vi "PathPlanner_GeomUtil_CubicLerp.vi"(6 "T":dbl, 8 "D":T1 {"Y" format="%14.3f"; "X" format="%14.3f"}, 9 "C":T1 {"Y" format="%14.3f"; "X" format="%14.3f"}, 10 "B":T1 {"Y" format="%14.3f"; "X" format="%14.3f"}, 11 "A":T1 {"Y" format="%14.3f"; "X" format="%14.3f"}) -> (3 "Lerp":T1 {"Y" format="%14.3f"; "X" format="%14.3f"})   [LabVIEW 2019, in "PathPlanner24.lvlib"]
doc: "Cubic interpolation between Translation2ds\n \nInputs: \n - a - translation2d - Position 1\n - b - translation2d - Position 2\n - c - translation2d - Position 3\n - t - double - Interpolation factor (0.0-1.0)\n\nOutputs:\n - Lerp - translation2d - Interpolated value"
uses:
  PathPlanner24.lvlib
  <vilib>/Rock Robotics/WPI/ThirdParty/JAS_Junk/TrajLib/TypeDef/TRANSLATION2D.ctl
  <vilib>/Rock Robotics/WPI/ThirdParty/JAS_Junk/TrajLib/Trajectory_Library.lvlib
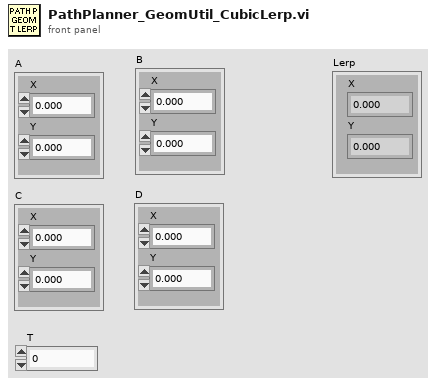
[diagram p1: front panel]
types:
  T1 = typedef "Trajectory_Library.lvlib/TRANSLATION2D.ctl" = cluster{"X":dbl, "Y":dbl}
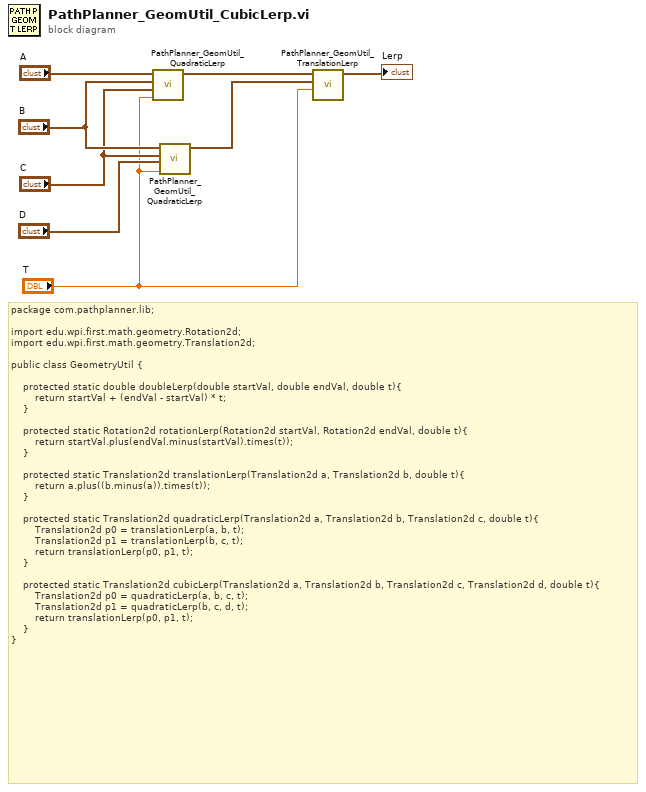
[diagram p0: block diagram]
diagram:
  # "package com.pathplanner.lib;\n\nimport edu.wpi.first.math.geometry.Rotation2d;\nimport edu.wpi.first.math.geometry.Translation2d;\n\npublic class GeometryUtil {\n\n    protected static double doubleLerp(double startVal, double endVal, double t){\n        return startVal + (endVal - startVal) * t;\n    }\n\n    protected static Rotation2d rotationLerp(Rotation2d startVal, Rotation2d endVal, double t){\n        return startVal.plus(endVal.minus(startVal).times(t));\n    }\n\n    protected static Translation2d translationLerp(Translation2d a, Translation2d b, double t){\n        return a.plus((b.minus(a)).times(t));\n    }\n\n    protected static Translation2d quadraticLerp(Translation2d a, Translation2d b, Translation2d c, double t){\n        Translation2d p0 = translationLerp(a, b, t);\n        Translation2d p1 = translationLerp(b, c, t);\n        return translationLerp(p0, p1, t);\n    }\n\n    protected static Translation2d cubicLerp(Translation2d a, Translation2d b, Translation2d c, Translation2d d, double t){\n        Translation2d p0 = quadraticLerp(a, b, c, t);\n        Translation2d p1 = quadraticLerp(b, c, d, t);\n        return translationLerp(p0, p1, t);\n    }\n}"
  n1 = call "PathPlanner_GeomUtil_QuadraticLerp.vi"("T"="T", "C"="C", "B"="B", "A"="A") -> ("Lerp"=w2:T1)  [unwired: 7 in]
  n2 = call "PathPlanner_GeomUtil_QuadraticLerp.vi"("T"="T", "C"="D", "B"="C", "A"="B") -> ("Lerp"=w1:T1)  [unwired: 7 in]
  n3 = call "PathPlanner_GeomUtil_TranslationLerp.vi"("T"="T", "EndVal"=w1, "StartVal"=w2) -> ("Lerp"=→"Lerp":T1)  [unwired: 8 in]
